vi "Get cif_manager_PluginTypeReply.vi"(8 "error in (no error)":errorcluster, 11 "gRPCid":T1) -> (0 "error out":errorcluster, 2 "package_templatemessage":T2, 3 "gRPCid out":T1)   [LabVIEW 2021, in "CIF_Manager_server.lvlib"]
uses:
  CIF_Manager_server.lvlib
  cif_manager_PluginTypeReply.ctl
  cif_manager_PluginType.ctl
  cif_manager_PluginVersion.ctl
  cif_manager_Error.ctl
  <vilib>/gRPC/LabVIEW gRPC Library/Shared/grpcId.ctl
  cif_manager_PluginTypeReply_Flat.ctl
  cif_manager_PluginType_Flat.ctl
  cif_manager_PluginVersion_Flat.ctl
  cif_manager_Error_Flat.ctl
  2ed25e12-861d-4677-8ead-ace2906b2041.vi
  <vilib>/gRPC/LabVIEW gRPC Library/Shared/TranslateGrpcError.vi
  FlatToRichcif_manager_PluginType.vi
  FlatToRichcif_manager_Error.vi
  FlatToRichcif_manager_PluginVersion.vi
  <vilib>/gRPC/LabVIEW gRPC Library/Server API/Server/Get Server DLL Path.vi
  <vilib>/Utility/error.llb/Error Cluster From Error Code.vi
  <vilib>/gRPC/LabVIEW gRPC Library/grpc-lvsupport-release.lvlib
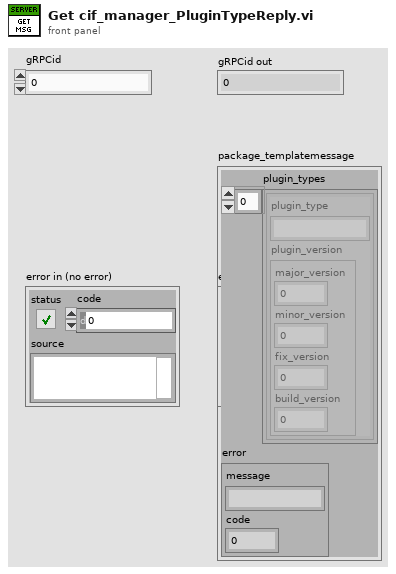
[diagram p1: front panel]
types:
  T1 = typedef "grpc-lvsupport-release.lvlib/grpcId.ctl" = u64
  T2 = typedef "CIF_Manager_server.lvlib/cif_manager_PluginTypeReply.ctl" = cluster{"plugin_types":T3[], "error":T5}
  T3 = typedef "CIF_Manager_server.lvlib/cif_manager_PluginType.ctl" = cluster{"plugin_type":string, "plugin_version":T4}
  T4 = typedef "CIF_Manager_server.lvlib/cif_manager_PluginVersion.ctl" = cluster{"major_version":i32, "minor_version":i32, "fix_version":i32, "build_version":i32}
  T5 = typedef "CIF_Manager_server.lvlib/cif_manager_Error.ctl" = cluster{"message":string, "code":i32}
  T6 = typedef "CIF_Manager_server.lvlib/cif_manager_PluginTypeReply_Flat.ctl" = cluster{"plugin_types":T7[], "error":T9}
  T7 = typedef "CIF_Manager_server.lvlib/cif_manager_PluginType_Flat.ctl" = cluster{"plugin_type":string, "plugin_version":T8}
  T8 = typedef "CIF_Manager_server.lvlib/cif_manager_PluginVersion_Flat.ctl" = cluster{"major_version":i32, "minor_version":i32, "fix_version":i32, "build_version":i32}
  T9 = typedef "CIF_Manager_server.lvlib/cif_manager_Error_Flat.ctl" = cluster{"message":string, "code":i32}
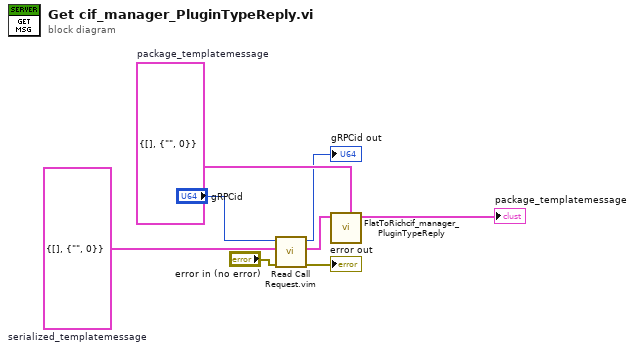
[diagram p0: block diagram]
diagram:
  w6 = T6 {"plugin_types"=[], "error"={"message"="", "code"=0}}  # serialized_templatemessage
  w5 = T2 {"plugin_types"=[], "error"={"message"="", "code"=0}}  # package_templatemessage
  n1 = call "Read Call Request.vim"("error in"="error in (no error)", "Request Type"=w6, "gRPCid in"="gRPCid") -> ("error out"=→"error out":errorcluster, "Request Data"=w4:T6, "gRPCid out"=→"gRPCid out":T1)  [unwired: 6 in]
  n2 = call "FlatToRichcif_manager_PluginTypeReply.vi"("OutputClusterType"=w5, "InputCluster"=w4) -> ("OutputCluster"=→"package_templatemessage":T2)  [unwired: 9 in]
